vi "Translate tag locations.vi"() -> ()   [LabVIEW 2023]
panel:
  out "tag info":dbl[][](array[numeric])
  out "output array":string[][](array[string])
  in  "Array":string[](array[string])=["1", "593.68", "9.68", "53.38", "120°", "2", "637.21", "34.79", "53.38", "120°", "3", "652.73", "196.17", "57.13", "180°", "4", "652.73", "218.42", "57.13", "180°", "5", "578.77", "323.00", "53.38", "270°", "6", "72.5", "323.00", "53.38", "270°", "7", "-1.50", "218.42", "57.13", "0°", "8", "-1.50", "196.17", "57.13", "0°", "9", "14.02", "34.79", "53.38", "60°", "10", "57.54", "9.68", "53.38", "60°", "11", "468.69", "146.19", "52.00", "300°", "12", "468.69", "177.10", "52.00", "60°", "13", "441.74", "161.62", "52.00", "180°", "14", "209.48", "161.62", "52.00", "0°", "15", "182.73", "177.10", "52.00", "120°", "16", "182.73", "146.19", "52.00", "240°"]
  # "29.1933"
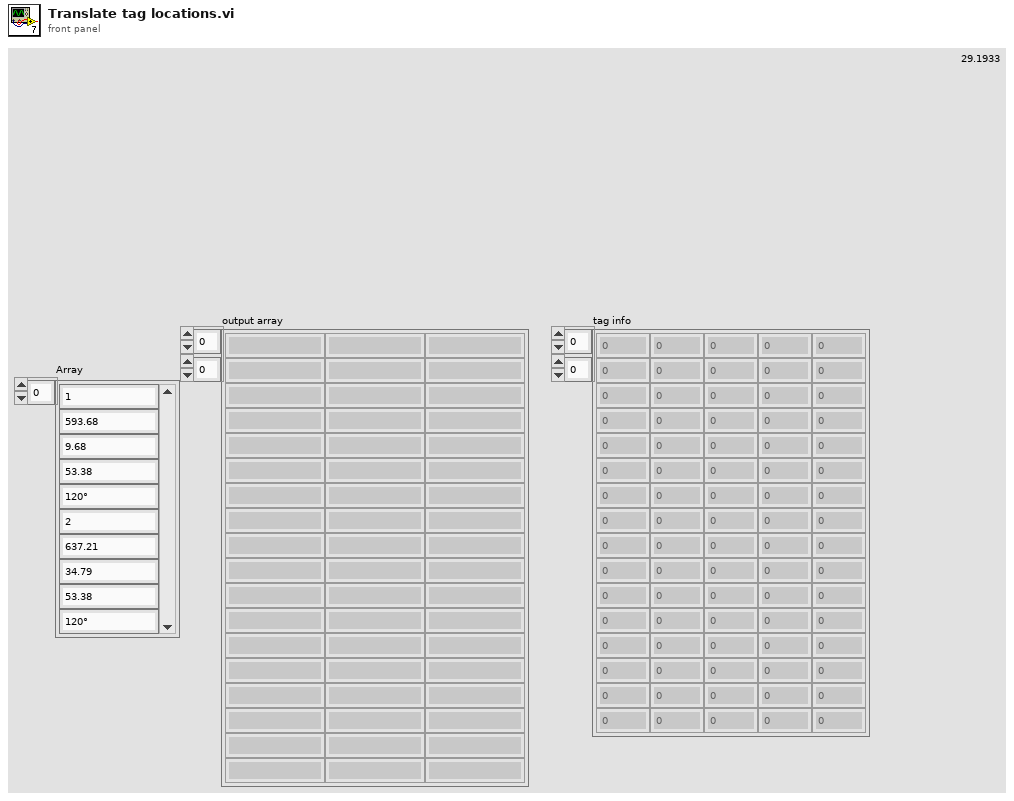
[diagram p1: front panel]
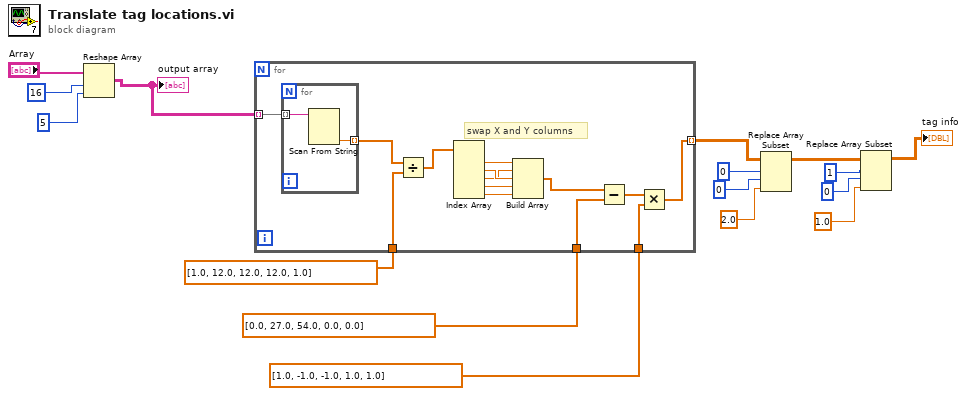
[diagram p0: block diagram]
diagram:
  n1 = Reshape Array("Array", 16 ("dimension size"), 5 ("dimension size")) -> (w13:string[][])
  "output array" <- w13
  n2 = for {
    tunnel: w13 -> [w30] mode=indexing
    tunnel: [w17] -> w9 mode=indexing
    tunnel: dbl[] [1.0, 12.0, 12.0, 12.0, 1.0] ("y") -> [w28]
    tunnel: dbl[] [0.0, 27.0, 54.0, 0.0, 0.0] ("y") -> [w27]
    tunnel: dbl[] [1.0, -1.0, -1.0, 1.0, 1.0] ("y") -> [w25]
    # "swap X and Y columns"
    n3 = for {
      tunnel: w30 -> [w32] mode=indexing
      tunnel: [w31] -> w29 mode=indexing
      n4 = Scan From String(input string=w32) -> (output 1=w31:dbl)  [unwired: 4 in, 3 out]
    }
    n5 = Divide(x=w29, y=w28) -> (x/y=w19:dbl[])
    n6 = Index Array(array=w19) -> (element #1=w24:dbl, element #2=w23:dbl, element #3=w22:dbl, element #4=w21:dbl, element #5=w20:dbl)  [unwired: 5 in]
    n7 = Build Array(w24, w22, w23, w21, w20) -> (w18:dbl[])
    n8 = Subtract(x=w18, y=w27) -> (x-y=w26:dbl[])
    n9 = Multiply(x=w26, y=w25) -> (x*y=w17:dbl[])
  }
  n10 = Replace Array Subset(array=w9, new element=2.0 ("new element/subarray"), index (row)=0, index (col)=0) -> (w5:dbl[][])
  n11 = Replace Array Subset(array=w5, new element=1.0 ("new element/subarray"), index (row)=1, index (col)=0) -> (→"tag info":dbl[][])
